vi "Init Comms.vi"(8 "error in (no error)":errorcluster, 11 "Communications in":refnum<class "Communications.lvclass">) -> (0 "error out":errorcluster, 3 "Communications out":refnum<class "Communications.lvclass">)   [LabVIEW 2016, in "Communications.lvclass"]
uses:
  Communications.lvclass
  C:/Program Files (x86)/National Instruments/LabVIEW 2016/vi.lib/ActorFramework/Actor/Actor.lvclass
  Communications.lvclass/Communications.ctl
  <vilib>/ActorFramework/Actor/Actor.lvclass/Actor.ctl
  <vilib>/ActorFramework/Message Enqueuer/Message Enqueuer.lvclass/Message Enqueuer.ctl
  Template Module Messages/Subscribe Request Msg/Subscribe Request Msg.lvclass/Subscribe Request Msg.ctl
  Read Communications Configuration.vi
  <vilib>/ActorFramework/Message Enqueuer/Init from Existing Queue.vi
  <vilib>/ActorFramework/Message Enqueuer/Enqueue.vi
  Template Module Messages/Subscribe Request Msg/Subscribe Request Msg.lvclass
  C:/Program Files (x86)/National Instruments/LabVIEW 2016/vi.lib/ActorFramework/Message/Message.lvclass
  <vilib>/ActorFramework/Message Priority Queue/Priority Enqueue.vi
  <vilib>/ActorFramework/Message Enqueuer/Message Enqueuer.lvclass
  <vilib>/ActorFramework/Actor/Actor.lvclass
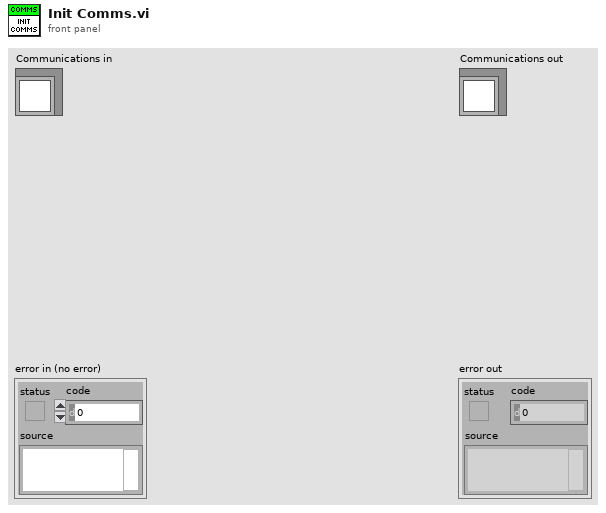
[diagram p1: front panel]
types:
  T1 = typedef "Communications Configuration.ctl" = cluster{"Subscribe to modules":string[]}
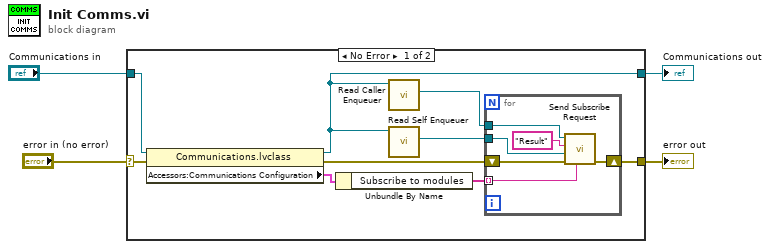
[diagram p0: block diagram]
diagram:
  n1 = case shown="No Error" "error in (no error)" {
    selector: "error in (no error)" -> [w13 w21]
    tunnel: [w7 w21] -> w3
    tunnel: [w6 w20] -> w1
    tunnel: "Communications in" -> [w12 w20]
    frame No Error {
      n2 = property class="Communications.lvclass"(reference=w12, error in=w13) -> (reference out=w6:refnum<class "Communications.lvclass">, error out=w8:errorcluster, "Accessors:Communications Configuration"=w11:T1)
      n3 = Unbundle By Name(w11) -> ("Subscribe to modules"=w10:string[])
      n4 = call <vilib>:"Read Caller Enqueuer.vi"("Actor"=w6) -> ("Caller Enqueuer"=w9:refnum<class "Message Enqueuer.lvclass">)  [unwired: 10 in]
      n5 = call <vilib>:"Read Self Enqueuer.vi"("Actor"=w6) -> ("Self Enqueuer"=w5:refnum<class "Message Enqueuer.lvclass">)  [unwired: 10 in]
      n6 = for {
        tunnel: w10 -> [w14] mode=indexing
        tunnel: w9 -> [w19]
        shift-right: [w16] -> w7
        shift-left: w8 -> [w17]
        tunnel: w5 -> [w15]
        n7 = call "Send Subscribe Request.vi"("Broadcaster"=w14, "error in (no error)"=w17, "Subscriber Enqueuer"=w15, "Topic"="Result", "Message Enqueuer"=w19) -> ("error out"=w16:errorcluster)  [unwired: 5 in, 1 out]
      }
    }
    frame Error {
    }
  }
  "error out" <- w3
  "Communications out" <- w1
